vi "MenuActive.vi"(11 "菜单引用":refnum<k9>) -> ()   [LabVIEW 2016]
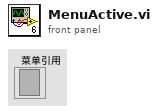
[diagram p1: front panel]
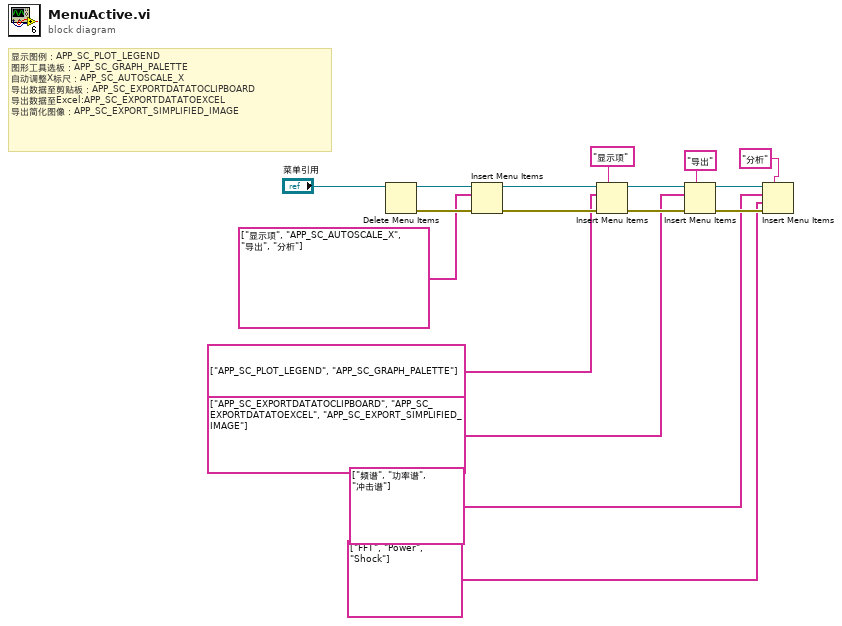
[diagram p0: block diagram]
diagram:
  # "显示图例：APP_SC_PLOT_LEGEND\n图形工具选板：APP_SC_GRAPH_PALETTE\n自动调整X标尺：APP_SC_AUTOSCALE_X\n导出数据至剪贴板：APP_SC_EXPORTDATATOCLIPBOARD\n导出数据至Excel:APP_SC_EXPORTDATATOEXCEL\n导出简化图像：APP_SC_EXPORT_SIMPLIFIED_IMAGE"
  n1 = Delete Menu Items(9:"菜单引用") -> (0:w15:errorcluster, 3:w16:refnum<k9>)  [unwired: 3 in]
  n2 = Insert Menu Items(6:w15, 8:string[] ["显示项", "APP_SC_AUTOSCALE_X", "导出", "分析"], 9:w16) -> (0:w12:errorcluster, 3:w13:refnum<k9>)  [unwired: 3 in, 1 out]
  n3 = Insert Menu Items(5:"显示项" ("菜单标识符"), 6:w12, 8:string[] ["APP_SC_PLOT_LEGEND", "APP_SC_GRAPH_PALETTE"], 9:w13) -> (0:w8:errorcluster, 3:w9:refnum<k9>)  [unwired: 2 in, 1 out]
  n4 = Insert Menu Items(5:"导出" ("菜单标识符"), 6:w8, 8:string[] ["APP_SC_EXPORTDATATOCLIPBOARD", "APP_SC_EXPORTDATATOEXCEL", "APP_SC_EXPORT_SIMPLIFIED_IMAGE"], 9:w9) -> (0:w4:errorcluster, 3:w5:refnum<k9>)  [unwired: 2 in, 1 out]
  n5 = Insert Menu Items(5:"分析" ("菜单标识符"), 6:w4, 7:string[] ["FFT", "Power", "Shock"], 8:string[] ["频谱", "功率谱", "冲击谱"], 9:w5) -> ()  [unwired: 1 in, 3 out]
